vi "Layer2_AckAnyPackets.vi"(0 "Serial Port to Use":refnum<visa-resource-name>="COM8", 11 "Error In":errorcluster) -> (4 "Serial Port to Use (out)":refnum<visa-resource-name>, 6 "A Packet Acked":bool, 8 "Ack Received":bool, 10 "Layer2 Payload":string, 15 "Error Out":errorcluster)   [LabVIEW 2012]
uses:
  Arduino_Serial_GlobalConstants.vi
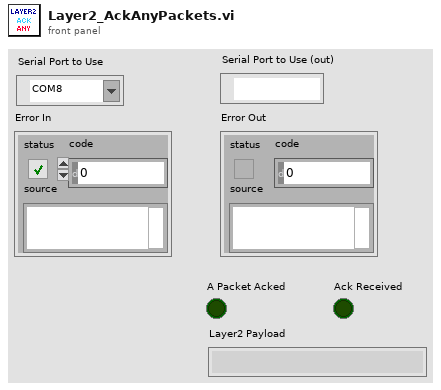
[diagram p1: front panel]
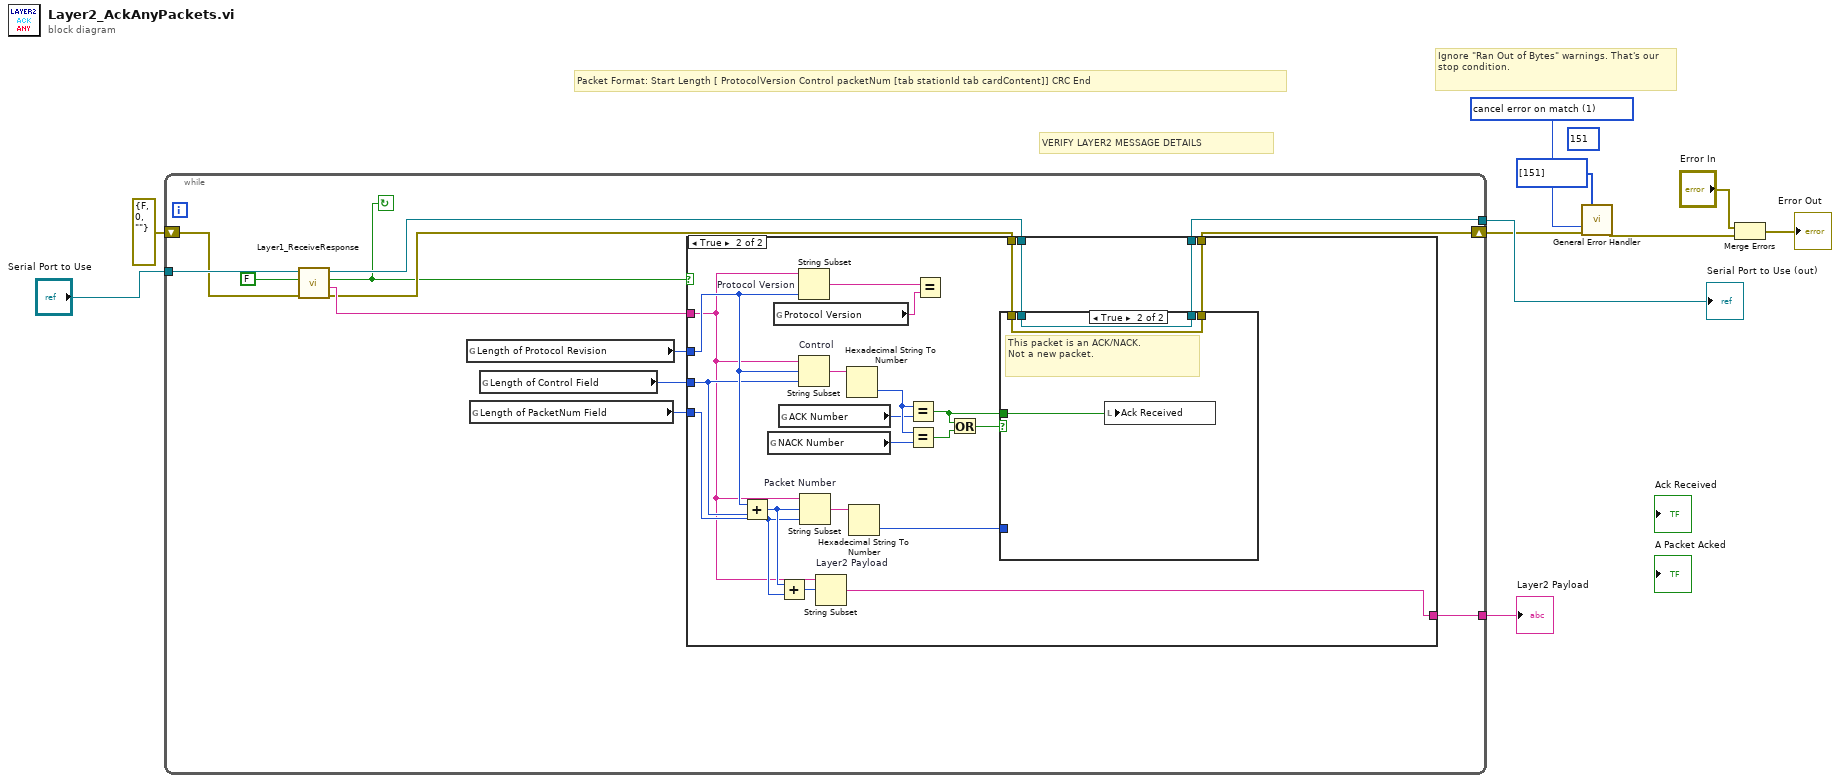
[diagram p0: block diagram]
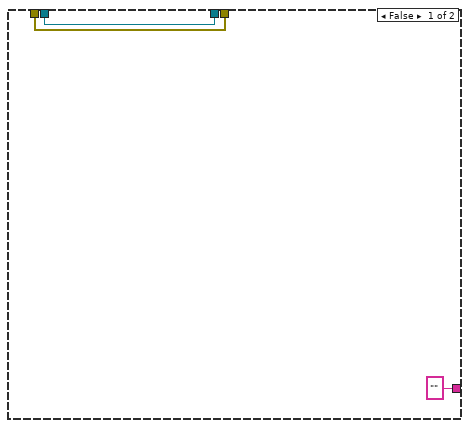
[diagram p2: hidden frame]
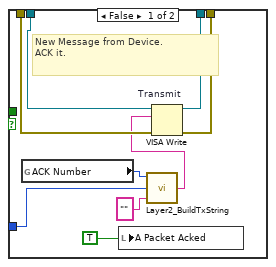
[diagram p3: hidden frame]
diagram:
  (unwired) 151 ("[exception code]")
  w7 = 1 items=["no exception", "cancel error on match", "set error on match"] ("[exception action] (none:0)")
  # "Ignore \"Ran Out of Bytes\" warnings. That's our stop condition."
  # "Packet Format: Start Length [ ProtocolVersion Control packetNum [tab stationId tab cardContent]] CRC End"
  # "VERIFY LAYER2 MESSAGE DETAILS"
  n1 = while {
    tunnel: "Serial Port to Use" -> [w23]
    tunnel: [w21] -> w9
    shift-right: [w12] -> w6
    shift-left: errorcluster {"status"=FALSE, "code"=0, "source"=""} ("Error Out") -> [w22]
    tunnel: [w13] -> w8
    stop <- w11 continue-if-true
    n2 = call "Layer1_ReceiveResponse.vi"("Error In"=w22, "Close Port After?"=FALSE, "Serial Port to Use (In)"=w23) -> ("Error Out"=w14:errorcluster, "Layer1 Payload"=w16:string, "Layer 1 Valid Packet"=w11:bool, "Serial Port to Use (out)"=w15:refnum<visa-resource-name>)  [unwired: 3 in, 2 out]
    n3 = global read "Arduino_Serial_GlobalConstants.vi" "Length of Protocol Revision"() -> (w18:i32)
    n4 = global read "Arduino_Serial_GlobalConstants.vi" "Length of PacketNum Field"() -> (w20:i32)
    n5 = global read "Arduino_Serial_GlobalConstants.vi" "Length of Control Field"() -> (w19:i32)
    n6 = case shown="True" w11 {
      tunnel: w16 -> [_ w40]
      tunnel: ["" ("read buffer") w27] -> w21
      tunnel: w20 -> [_ w42]
      tunnel: w19 -> [_ w45]
      tunnel: w18 -> [_ w46]
      tunnel: w14 -> [w24 w33]
      tunnel: w15 -> [w25 w32]
      tunnel: [w25 w31] -> w13
      tunnel: [w24 w30] -> w12
      frame False {
      }
      frame True {
        n7 = Add(x=w46, y=w45) -> (x+y=w43:i32)
        n8 = global read "Arduino_Serial_GlobalConstants.vi" "NACK Number"() -> (w36:i32)
        n9 = global read "Arduino_Serial_GlobalConstants.vi" "Protocol Version"() -> (w47:string)
        n10 = global read "Arduino_Serial_GlobalConstants.vi" "ACK Number"() -> (w37:i32)
        n11 = Add(x=w43, y=w42) -> (x+y=w41:i32)
        n12 = String Subset "Protocol Version"(string=w40, length (rest)=w46) -> (substring=w48:string)  [unwired: 1 in]
        n13 = String Subset "Control"(string=w40, offset (0)=w46, length (rest)=w45) -> (substring=w39:string)
        n14 = String Subset "Packet Number"(string=w40, offset (0)=w43, length (rest)=w42) -> (substring=w44:string)
        n15 = String Subset "Layer2 Payload"(string=w40, offset (0)=w41) -> (substring=w27:string)  [unwired: 1 in]
        n16 = Hexadecimal String To Number(string=w39) -> (number=w38:u32)  [unwired: 2 in, 1 out]
        n17 = Hexadecimal String To Number(string=w44) -> (number=w29:u32)  [unwired: 2 in, 1 out]
        n18 = Equal?(x=w38, y=w37) -> (x = y?=w28:bool)
        n19 = Equal?(x=w38, y=w36) -> (x = y?=w35:bool)
        n20 = Equal?(x=w48, y=w47) -> ()  [unwired: 1 out]
        n21 = Or(x=w28, y=w35) -> (x .or. y?=w34:bool)
        n22 = case shown="True" w34 {
          tunnel: w33 -> [w52 w59]
          tunnel: w32 -> [w53 w60]
          tunnel: [w51 w60] -> w31
          tunnel: [w50 w59] -> w30
          tunnel: w29 -> [w56 _]
          tunnel: w28 -> [_ w58]
          frame False {
            # "New Message from Device.\nACK it."
            n23 = global read "Arduino_Serial_GlobalConstants.vi" "ACK Number"() -> (w54:i32)
            n24 = local write "A Packet Acked"(TRUE ("Response Received")) -> ()
            n25 = call "Layer2_BuildTxString.vi"("Message"="", "PacketNum"=w56, "Control"=w54) -> ("Write Buffer"=w49:string)
            n26 = VISA Write "Transmit"(VISA resource name=w53, write buffer=w49, error in (no error)=w52) -> (VISA resource name out=w51:refnum<visa-resource-name>, error out=w50:errorcluster)  [unwired: 1 out]
          }
          frame True {
            # "This packet is an ACK/NACK.\nNot a new packet."
            n27 = local write "Ack Received"(w58) -> ()
          }
        }
      }
    }
  }
  "Layer2 Payload" <- w9
  "Serial Port to Use (out)" <- w8
  n28 = call <vilib>:"General Error Handler.vi"("[user-defined codes]"=i32[] [151], "type of dialog (OK msg:1)"=w7, "error in (no error)"=w6) -> ("error out"=w3:errorcluster)  [unwired: 8 in, 4 out]
  n29 = Merge Errors("Error In", w3) -> (→"Error Out":errorcluster)
